vi "Write Request.vi"(8 "error in (no error)":errorcluster, 10 "Request":bool, 11 "Elevator Controller Actor in":refnum<class "Elevator Controller Actor.lvclass">) -> (0 "error out":errorcluster, 3 "Elevator Controller Actor out":refnum<class "Elevator Controller Actor.lvclass">)   [LabVIEW 2019, in "Elevator Controller Actor.lvlib" / "Elevator Controller Actor.lvclass"]
uses:
  Elevator Controller Actor.lvclass
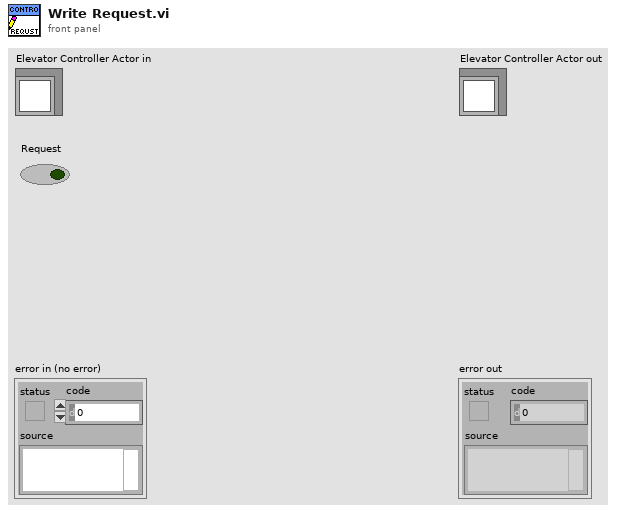
[diagram p1: front panel]
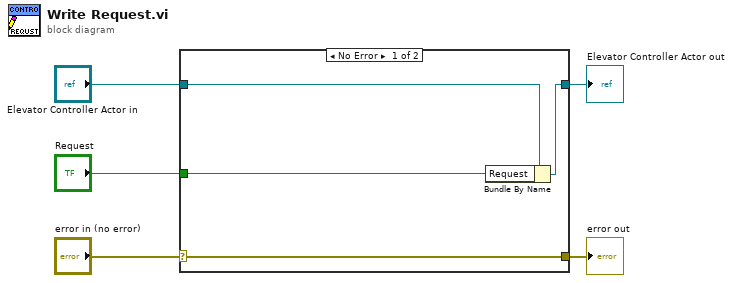
[diagram p0: block diagram]
diagram:
  n1 = case shown="No Error" "error in (no error)" {
    selector: "error in (no error)" -> [w9 w10]
    tunnel: [w9 w10] -> w4
    tunnel: [w7 w11] -> w2
    tunnel: "Elevator Controller Actor in" -> [w8 w11]
    tunnel: "Request" -> [w6 _]
    frame No Error {
      n2 = Bundle By Name(cluster=w8, "Request"=w6) -> (w7:refnum<class "Elevator Controller Actor.lvclass">)
    }
    frame Error {
    }
  }
  "error out" <- w4
  "Elevator Controller Actor out" <- w2
